vi "parse -- split on regexp.vi"(7 "regexp":string="(\\s*[\\d\\.\\+\\-]+)+\\s*\\r?", 11 "string array":string[](array[string])=["eee d", "4", "12 34.0 56", "1 23 4", "yy uu iii oo"]) -> (0 "last line":string="4", 1 "after":string[](array[string])=["12 34.0 56", "1 23 4", "yy uu iii oo"], 2 "matching lines":string[](array[string])=["eee d"])   [LabVIEW 2014]
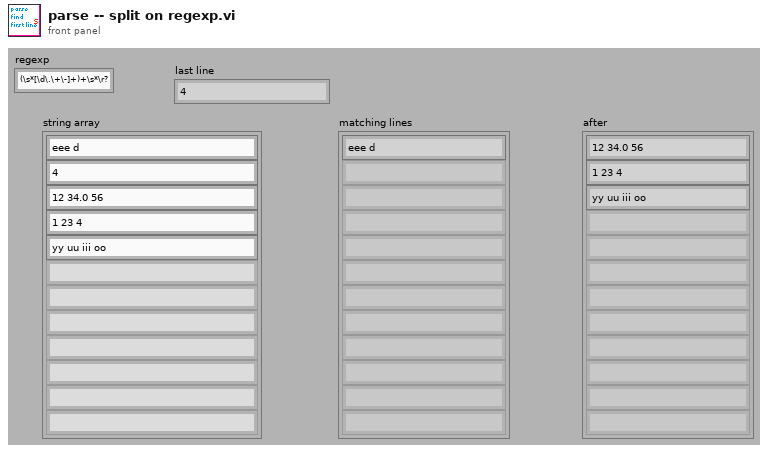
[diagram p1: front panel]
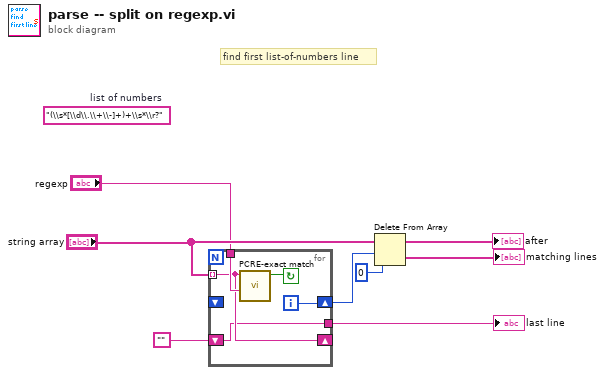
[diagram p0: block diagram]
diagram:
  (unwired) "(\\s*[\\d\\.\\+\\-]+)+\\s*\\r?"  # list of numbers
  # "find first list-of-numbers line"
  n1 = for {
    tunnel: "string array" -> [w10] mode=indexing
    shift-right: [w12] -> w4
    shift-left: _ -> [_]
    tunnel: "regexp" -> [w11]
    shift-right: [w10] -> _
    shift-left: "" -> [w9]
    tunnel: [w9] -> w1
    i -> [w12]
    stop <- w13 continue-if-true
    n2 = call "PCRE-exact match.vi"("regular expression"=w11, "input string"=w10) -> ("exact match"=w13:bool)  [unwired: 7 in, 2 out]
  }
  "last line" <- w1
  n3 = Delete From Array(array="string array", length=w4, index=0 ("index (row)")) -> (deleted portion=→"matching lines":string[], array with subset deleted=→"after":string[])
